vi "Example_Read.vi"() -> ()   [LabVIEW 2021]
panel:
  out "Waveform Graph":waveform(i32)[](graph)
  out "size (in bytes)":i64
  in  "Slide":i32(slide) scale=0.0..99.0
  in  "file path (use dialog)":path
  in  "stop":bool
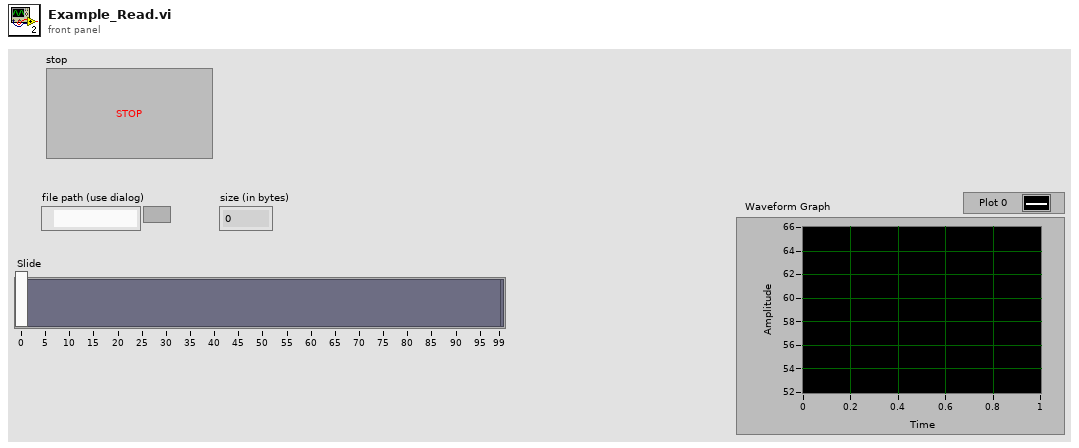
[diagram p1: front panel]
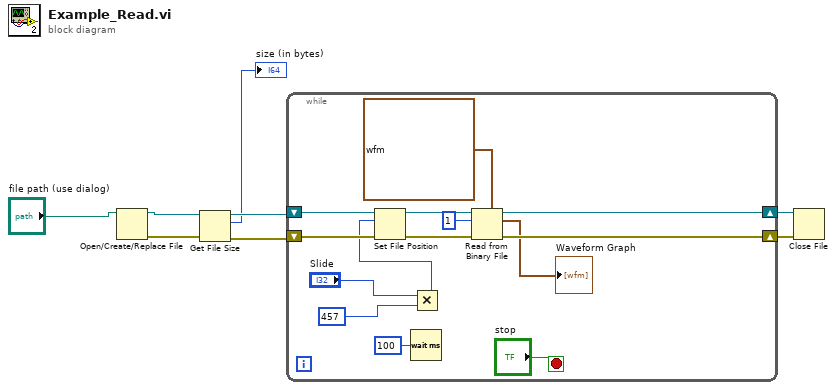
[diagram p0: block diagram]
diagram:
  n1 = Open/Create/Replace File(file path (use dialog)="file path (use dialog)") -> (refnum out=w5:refnum<file>, error out=w3:errorcluster)  [unwired: 5 in, 1 out]
  n2 = Get File Size(file=w5, error in=w3) -> (refnum out=w4:refnum<file>, size (in bytes)=→"size (in bytes)":i64, 0:w2:errorcluster)
  n3 = while {
    shift-right: [w19] -> w8
    shift-left: w4 -> [w21]
    shift-right: [w18] -> w7
    shift-left: w2 -> [w20]
    stop <- "stop" stop-if-true
    n4 = Wait (ms)(milliseconds to wait=u32 100) -> ()  [unwired: 1 out]
    n5 = Multiply(x="Slide", y=457) -> (x*y=w11:i32)
    n6 = Set File Position(offset (in bytes) (0)=w11, refnum=w21) -> (refnum out=w12:refnum<file>)  [unwired: 2 in, 1 out]
    n7 = Read from Binary File(5:waveform(i32) {"t0"=timestamp(0 s since 1904-01-01), "dt"=1.0, "Y"=[]} ("output waveform"), 8:w20, 10:1 ("count (1)"), 11:w12) -> (0:w18:errorcluster, 2:→"Waveform Graph":waveform(i32)[], 3:w19:refnum<file>)  [unwired: 2 in, 1 out]
  }
  n8 = Close File(refnum=w8, error in=w7) -> ()  [unwired: 2 out]
